vi "Send Disconnect.vi"(8 "error in (no error)":errorcluster, 11 "TCP Receive in":refnum<class "TCP Receive.lvclass">) -> (0 "error out":errorcluster, 3 "TCP Receive out":refnum<class "TCP Receive.lvclass">)   [LabVIEW 2020, in "TCP Receive.lvclass"]
uses:
  TCP Receive.lvclass
  <vilib>/addons/_Workers/Library/Classes/Message/Message.lvclass
  <vilib>/addons/_Workers/Library/Classes/Message/Enqueue Message to Queue.vi
  C:/Program Files (x86)/National Instruments/LabVIEW 2020/vi.lib/addons/_Workers/Library/Classes/Worker User/Worker User.lvclass
  C:/Program Files (x86)/National Instruments/LabVIEW 2020/vi.lib/addons/_Workers/Library/Classes/Worker/Worker.lvclass
  C:/Program Files (x86)/National Instruments/LabVIEW 2020/vi.lib/addons/_Workers/Library/Classes/Workers Object/Workers Object.lvclass
  C:/Users/TestAdmin/git/TCP-Workers/Workers/TCP Receive/TCP Receive.lvclass
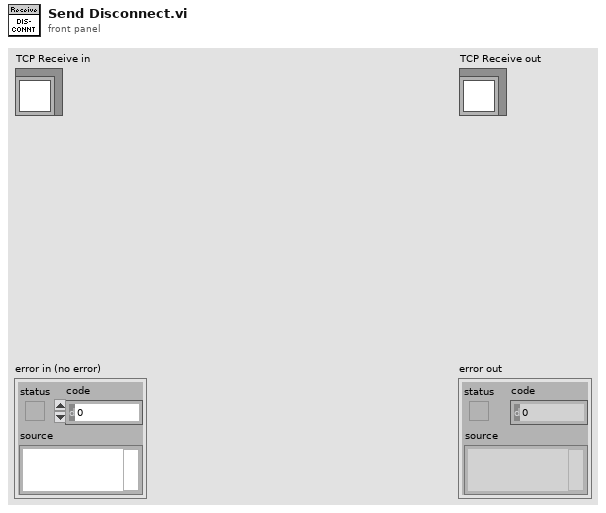
[diagram p1: front panel]
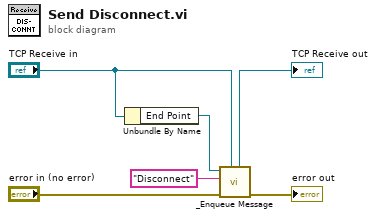
[diagram p0: block diagram]
diagram:
  n1 = Unbundle By Name("TCP Receive in") -> ("End Point"=w6:refnum<class "Message Queue.lvclass">)
  n2 = call-poly <vilib>:"_Enqueue Message.vi"("Worker"="TCP Receive in", "error in"="error in (no error)", "Case Label"="Disconnect", "Message Queue"=w6) -> ("error out"=→"error out":errorcluster, "dup Worker out"=→"TCP Receive out":refnum<class "TCP Receive.lvclass">)  [unwired: 5 in, 1 out]
